vi "connect.vi"(8 "error in (no error)":errorcluster, 11 "Electrometer in":refnum<class "Electrometer.lvclass">) -> (0 "error out":errorcluster, 2 "VISA resource name":refnum<visa-resource-name>, 3 "Electrometer out":refnum<class "Electrometer.lvclass">)   [LabVIEW 2016, in "Electrometer.lvclass"]
uses:
  Electrometer.lvclass
  <vilib>/Utility/error.llb/DialogType.ctl
  ElectrometerConfiguration/ElectrometerCOMConfiguration.lvclass
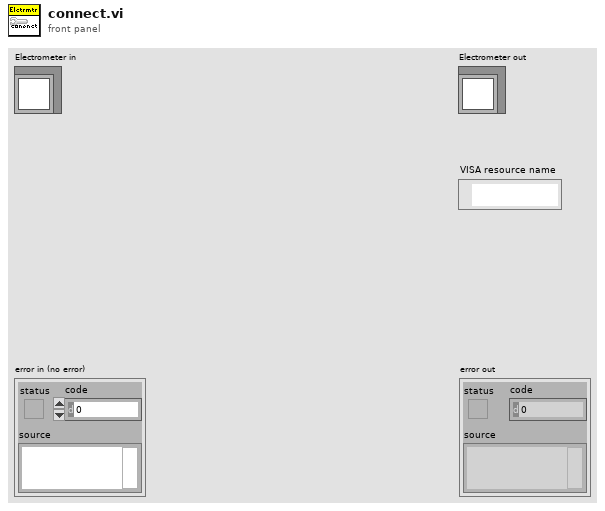
[diagram p1: front panel]
types:
  T1 = typedef "DialogType.ctl" = u16
  T2 = typedef "ElectrometerTypedefs.lvlib/termChar.ctl" = enum16{"CR", "CR+LF", "LF", "LF+CR"}
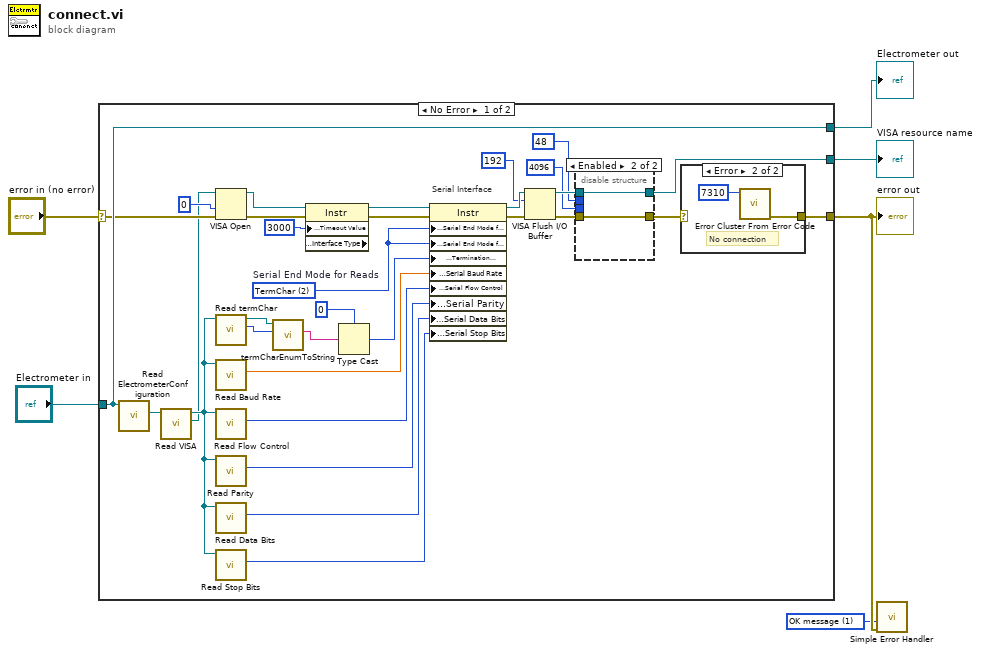
[diagram p0: block diagram]
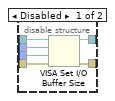
[diagram p2: hidden frame]
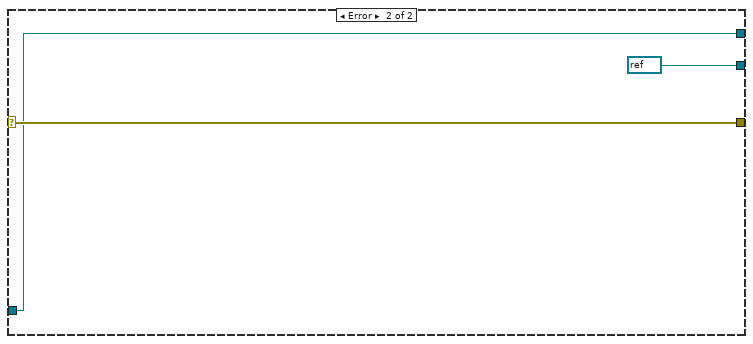
[diagram p4: hidden frame]
diagram:
  w1 = T1 1 items=["no dialog", "OK message", "continue or stop message", "OK message + warnings", "continue/stop + warnings"] ("type of dialog (OK msg:1)")
  n1 = case shown="No Error" "error in (no error)" {
    selector: "error in (no error)" -> [w20 w52]
    tunnel: [w11 w52] -> w2
    tunnel: [w29 w51] -> w4
    tunnel: "Electrometer in" -> [w29 w51]
    tunnel: [w23 refnum<visa-resource-name> refnum ("VISA resource name")] -> w3
    frame No Error {
      w30 = u16 2 items=["None", "LastBit", "TermChar"]  # Serial End Mode for Reads
      # "Serial Interface"
      n2 = call "Read ElectrometerConfiguration.vi"("Electrometer in"=w29) -> ("ElectrometerConfiguration"=w18:refnum<class "ElectrometerCOMConfiguration.lvclass">)  [unwired: 8 in, 2 out]
      n3 = call-dynamic "Read VISA.vi"("ElectrometerConfiguration in"=w18) -> ("VISA"=w16:refnum<visa-resource-name>, "ElectrometerConfiguration out"=w17:refnum<class "ElectrometerCOMConfiguration.lvclass">)  [unwired: 8 in, 1 out]
      n4 = VISA Open(access mode=u32 0, error in (no error)=w20, VISA resource name=w16) -> (VISA resource name=w21:refnum<visa-resource-name>, error out=w13:errorcluster)  [unwired: 2 in]
      n5 = call-dynamic "Read termChar.vi"("ElectrometerConfiguration in"=w17) -> ("termChar"=w9:T2, "ElectrometerConfiguration out"=w8:refnum<class "ElectrometerCOMConfiguration.lvclass">)  [unwired: 8 in, 1 out]
      n6 = call-dynamic "Read Baud Rate.vi"("ElectrometerConfiguration in"=w17) -> ("Baud Rate"=w25:dbl)  [unwired: 8 in, 2 out]
      n7 = call-dynamic "Read Flow Control.vi"("ElectrometerConfiguration in"=w17) -> ("Flow Control"=w26:u16)  [unwired: 8 in, 2 out]
      n8 = call-dynamic "Read Parity.vi"("ElectrometerConfiguration in"=w17) -> ("Parity"=w27:u16)  [unwired: 8 in, 2 out]
      n9 = call-dynamic "Read Data Bits.vi"("ElectrometerConfiguration in"=w17) -> ("Data Bits"=w24:u16)  [unwired: 8 in, 2 out]
      n10 = call-dynamic "Read Stop Bits.vi"("ElectrometerConfiguration in"=w17) -> ("Stop Bits"=w28:u16)  [unwired: 8 in, 2 out]
      n11 = call "termCharEnumToString.vi"("termChar"=w9, "ElectrometerCOMConfiguration in"=w8) -> ("termChar"=w7:string)  [unwired: 7 in, 2 out]
      n12 = property class="Instr" props=["General Settings:Timeout Value", "Interface Information:Interface Type"](reference=w21, error in=w13, "General Settings:Timeout Value"=u32 3000) -> (reference out=w15:refnum<visa-resource-name>, error out=w19:errorcluster)  [unwired: 1 out]
      n13 = Type Cast(type=u8 0, x=w7) -> (*(type *) &x=w10:u8)
      n14 = property class="Instr"(reference=w15, error in=w19, "Serial Settings:Serial End Mode for Reads"=w30, "Serial Settings:Serial End Mode for Writes"=w30, "Message Based Settings:Termination Character"=w10, "Serial Settings:Serial Baud Rate"=w25, "Serial Settings:Serial Flow Control"=w26, "Serial Settings:Serial Parity"=w27, "Serial Settings:Serial Data Bits"=w24, "Serial Settings:Serial Stop Bits"=w28) -> (reference out=w35:refnum<visa-resource-name>, error out=w37:errorcluster)
      n15 = VISA Flush I/O Buffer(VISA resource name=w35, mask (16)=u16 192, error in (no error)=w37) -> (VISA resource name out=w38:refnum<visa-resource-name>, error out=w36:errorcluster)
      n16 = disable-structure shown="Enabled" {
        disable-tunnel: w38 -> [w44 w46]
        disable-tunnel: w36 -> [w43 w45]
        disable-tunnel: u32 4096 ("size (0)") -> [w42 _]
        disable-tunnel: u16 48 ("mask (16)") -> [w41 _]
        disable-tunnel: [w40 w46] -> w23
        disable-tunnel: [w39 w45] -> w12
        frame Disabled {
          n17 = VISA Set I/O Buffer Size(VISA resource name=w44, mask (16)=w41, size (4096)=w42, error in (no error)=w43) -> (VISA resource name out=w40:refnum<visa-resource-name>, error out=w39:errorcluster)
        }
        frame Enabled {
        }
      }
      n18 = case shown="Error" w12 {
        selector: w12 -> [w47 _]
        tunnel: [w47 w49] -> w11
        frame No Error {
        }
        frame Error {
          # "No connection"
          n19 = call <vilib>:"Error Cluster From Error Code.vi"("error code (0)"=7310) -> ("error out"=w49:errorcluster)  [unwired: 8 in]
        }
      }
    }
    frame Error {
    }
  }
  "error out" <- w2
  "Electrometer out" <- w4
  "VISA resource name" <- w3
  n20 = call <vilib>:"Simple Error Handler.vi"("type of dialog (OK msg:1)"=w1, "error in (no error)"=w2) -> ()  [unwired: 3 in, 5 out]
